vi "buffered_waveform_chart.vi"() -> ()   [LabVIEW 2019]
panel:
  in  "stop":bool
  out "Waveform Chart":i32(graph)
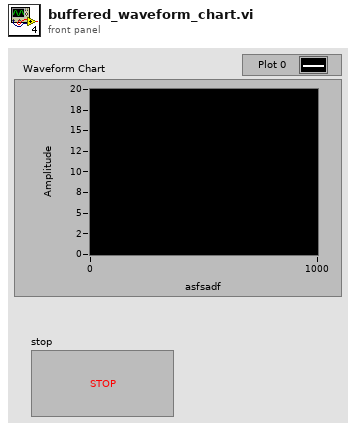
[diagram p1: front panel]
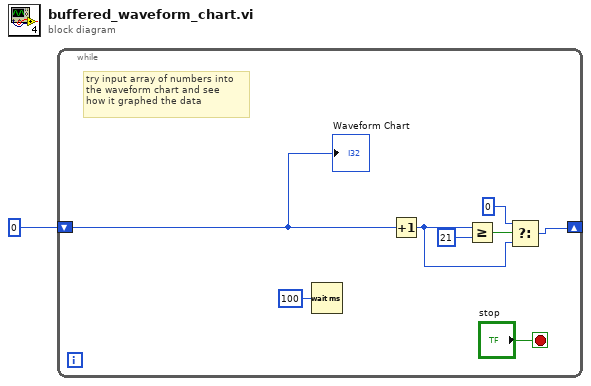
[diagram p0: block diagram]
diagram:
  n1 = while {
    shift-right: [w3] -> _
    shift-left: 0 -> [w2]
    stop <- "stop" stop-if-true
    # "try input array of numbers into\nthe waveform chart and see \nhow it graphed the data"
    n2 = Wait (ms)(milliseconds to wait=u32 100) -> ()  [unwired: 1 out]
    n3 = Increment(x=w2) -> (x+1=w4:i32)
    n4 = Greater Or Equal?(x=w4, y=21) -> (x >= y?=w6:bool)
    n5 = Select(t=0 ("y"), s=w6, f=w4) -> (s? t:f=w3:i32)
    "Waveform Chart" <- w2
  }
